vi "PH_4_Pos_Selector.Position Calculator.vi"(1 "Current Axes Positions":T1, 2 "Position Array":T1[](array[typedef])) -> (0 "Current Position":T2 items=["unknown", "Position I", "Position II", "Position III", "Position IV", "moving"])   [LabVIEW 2014, in "PH_4_Pos_Selector.lvlib"]
uses:
  PH_4_Pos_Selector.lvlib
  PH_4_Pos_Selector.Position Selector.ctl
  PH_4_Pos_Selector.Position.ctl
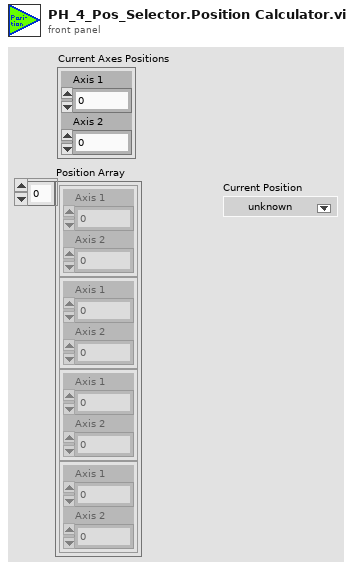
[diagram p1: front panel]
types:
  T1 = typedef "PH_4_Pos_Selector.lvlib/PH_4_Pos_Selector.Position.ctl" = cluster{"Axis 1":dbl, "Axis 2":dbl}
  T2 = typedef "PH_4_Pos_Selector.lvlib/PH_4_Pos_Selector.Position Selector.ctl" = u16
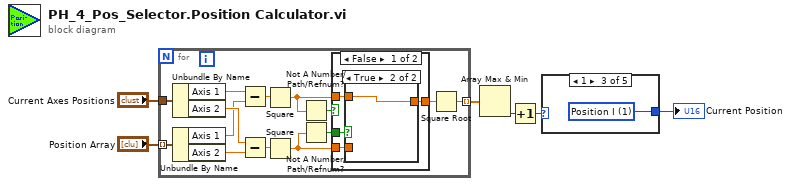
[diagram p0: block diagram]
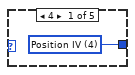
[diagram p2: hidden frame]
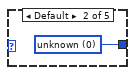
[diagram p3: hidden frame]
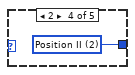
[diagram p4: hidden frame]
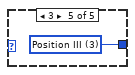
[diagram p5: hidden frame]
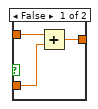
[diagram p6: hidden frame]
diagram:
  n1 = for {
    tunnel: "Current Axes Positions" -> [w20]
    tunnel: "Position Array" -> [w19] mode=indexing
    tunnel: [w14] -> w3 mode=indexing
    n2 = Unbundle By Name(w20) -> ("Axis 1"=w18:dbl, "Axis 2"=w17:dbl)
    n3 = Unbundle By Name(w19) -> ("Axis 1"=w13:dbl, "Axis 2"=w12:dbl)
    n4 = Subtract(x=w18, y=w13) -> (x-y=w15:dbl)
    n5 = Subtract(x=w17, y=w12) -> (x-y=w16:dbl)
    n6 = Square(x=w15) -> (x^2=w10:dbl)
    n7 = Square(x=w16) -> (x^2=w11:dbl)
    n8 = Not A Number/Path/Refnum?(number/path/refnum=w10) -> (NaN/Path/Refnum?=w8:bool)
    n9 = Not A Number/Path/Refnum?(number/path/refnum=w11) -> (NaN/Path/Refnum?=w7:bool)
    n10 = case shown="False" w8 {
      tunnel: w11 -> [w24 w29]
      tunnel: w10 -> [w23 _]
      tunnel: [w22 w29] -> w9
      tunnel: w7 -> [w21 _]
      frame False {
        n11 = case shown="True" w21 {
          tunnel: w24 -> [w27 _]
          tunnel: w23 -> [w26 w28]
          tunnel: [w25 w28] -> w22
          frame False {
            n12 = Add(x=w26, y=w27) -> (x+y=w25:dbl)
          }
          frame True {
          }
        }
      }
      frame True {
      }
    }
    n13 = Square Root(x=w9) -> (sqrt(x)=w14:dbl)
  }
  n14 = Array Max & Min(array=w3) -> (min index (indices)=w5:i32)  [unwired: 3 out]
  n15 = Increment(x=w5) -> (x+1=w6:i32)
  n16 = case shown="1" w6 {
    tunnel: [w30 w31 w32 w33 w34] -> w4
    frame 4 {
      w30 = T2 4 items=["unknown", "Position I", "Position II", "Position III", "Position IV"] ("Current Position")
    }
    frame Default {
      w31 = T2 0 items=["unknown", "Position I", "Position II", "Position III", "Position IV"] ("Current Position")
    }
    frame 1 {
      w32 = T2 1 items=["unknown", "Position I", "Position II", "Position III", "Position IV"] ("Current Position")
    }
    frame 2 {
      w33 = T2 2 items=["unknown", "Position I", "Position II", "Position III", "Position IV"] ("Current Position")
    }
    frame 3 {
      w34 = T2 3 items=["unknown", "Position I", "Position II", "Position III", "Position IV"] ("Current Position")
    }
  }
  "Current Position" <- w4
